vi "FailureLog.vi"(0 "Section":string, 2 "key":string, 5 "error in (no error)":errorcluster, 8 "Path":path) -> (19 "error out":errorcluster)   [LabVIEW 2009, in "MoAgSy.lvlib"]
uses:
  MoAgSy.lvlib
  <vilib>/Utility/config.llb/Write Key (String).vi
  <vilib>/Utility/config.llb/Write Key (I32).vi
  <vilib>/Utility/config.llb/Write Key (Boolean).vi
  <vilib>/Utility/config.llb/NI_LVConfig.lvlib
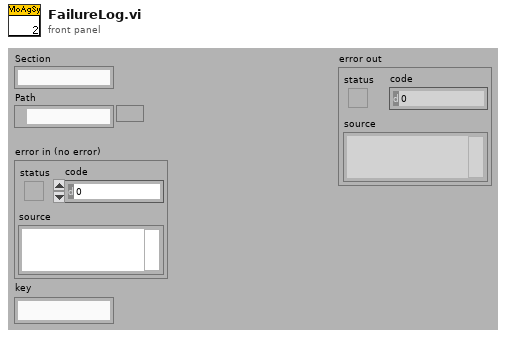
[diagram p1: front panel]
types:
  T1 = typedef "NI_LVConfig.lvlib/Config Data RefNum.ctl" = refnum<k1>
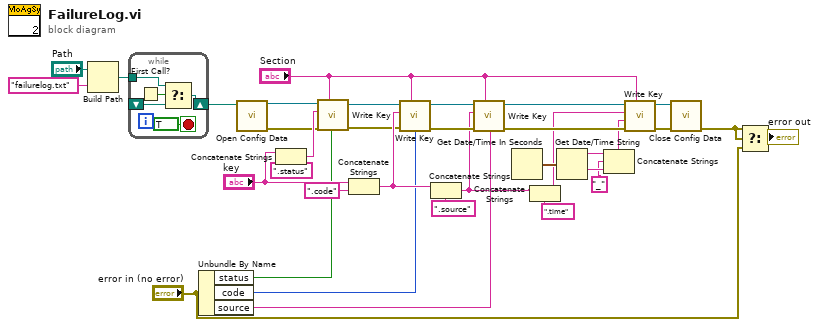
[diagram p0: block diagram]
diagram:
  n1 = Build Path(base path="Path", name or relative path="failurelog.txt") -> (appended path=w34:path)
  n2 = while {
    tunnel: w34 -> [w39]
    shift-right: [w38] -> w32
    shift-left: _ -> [w37]
    stop <- TRUE stop-if-true
    n3 = First Call?() -> (First Call?: T/F=w40:bool)
    n4 = Select(t=w39, s=w40, f=w37) -> (s? t:f=w38:path)
  }
  n5 = Unbundle By Name("error in (no error)") -> ("status"=w22:bool, "code"=w21:i32, "source"=w20:string)
  n6 = call <vilib>:"Open Config Data.vi"("configuration file path"=w32) -> ("error out"=w19:errorcluster, "refnum"=w31:T1)  [unwired: 8 in, 1 out]
  n7 = Concatenate Strings("key", ".status" ("string")) -> (w30:string)
  n8 = call-poly <vilib>:"Write Key.vi"("section"="Section", "error in (no error)"=w19, "value"=w22, "key"=w30, "refnum"=w31) -> ("error out"=w18:errorcluster, "refnum out"=w29:T1)  [unwired: 4 in, 1 out]
  n9 = Concatenate Strings("key", ".code" ("string")) -> (w24:string)
  n10 = call-poly <vilib>:"Write Key.vi"("section"="Section", "error in (no error)"=w18, "value"=w21, "key"=w24, "refnum"=w29) -> ("error out"=w17:errorcluster, "refnum out"=w25:T1)  [unwired: 4 in, 1 out]
  n11 = Concatenate Strings(w24, ".source" ("string")) -> (w2:string)
  n12 = call-poly <vilib>:"Write Key.vi"("section"="Section", "error in (no error)"=w17, "value"=w20, "key"=w2, "refnum"=w25) -> ("error out"=w11:errorcluster, "refnum out"=w13:T1)  [unwired: 4 in, 1 out]
  n13 = Get Date/Time In Seconds() -> (seconds since 1Jan1904=w8:timestamp)
  n14 = Concatenate Strings(w2, ".time" ("string")) -> (w1:string)
  n15 = Get Date/Time String(seconds (now)=w8) -> (date string=w7:string, time string=w6:string)  [unwired: 2 in]
  n16 = Concatenate Strings(w7, "_" ("string"), w6) -> (w4:string)
  n17 = call-poly <vilib>:"Write Key.vi"("section"="Section", "error in (no error)"=w11, "value"=w4, "key"=w1, "refnum"=w13) -> ("error out"=w10:errorcluster, "refnum out"=w12:T1)  [unwired: 4 in, 1 out]
  n18 = call <vilib>:"Close Config Data.vi"("error in (no error)"=w10, "refnum"=w12) -> ("error out"=w16:errorcluster)  [unwired: 8 in, 1 out]
  n19 = Select(t=w16, s=w16, f="error in (no error)") -> (s? t:f=→"error out":errorcluster)
